vi "AddressGroup.vi"(11 "Addresses":i32[](array[numeric])=[0, 246, 248, 250]) -> (3 "Group":cluster{"Tag'sIndex":i32[]}[](array[cluster]))   [LabVIEW 2020, in "ModBusCommon.lvlib"]
uses:
  ModBusCommon.lvlib
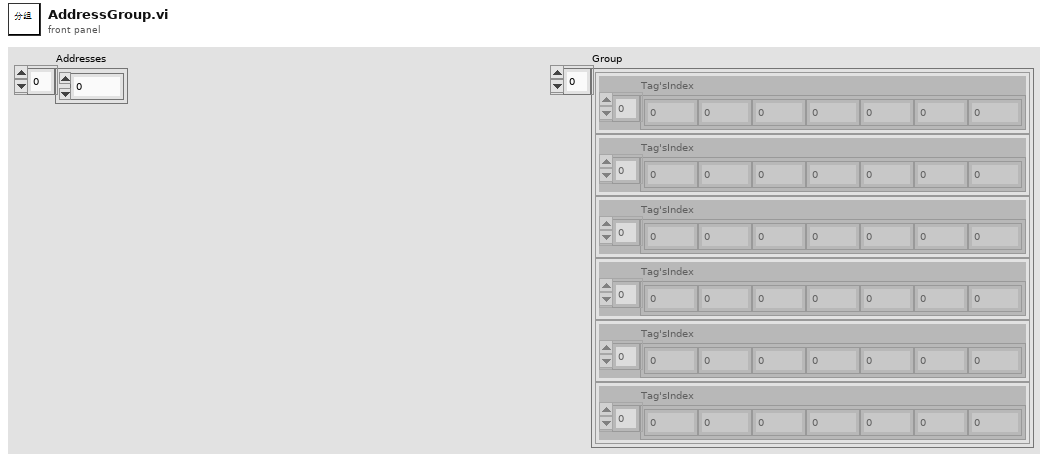
[diagram p1: front panel]
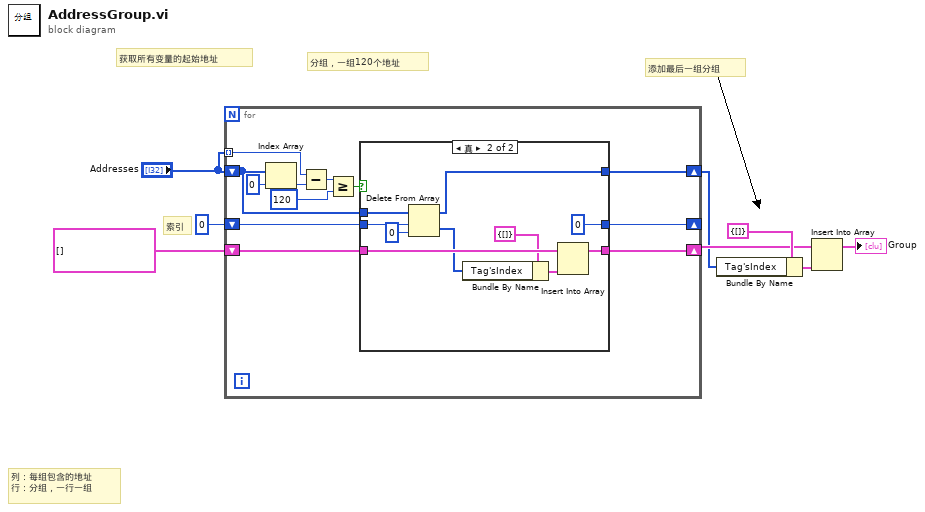
[diagram p0: block diagram]
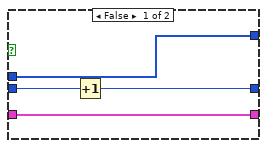
[diagram p2: hidden frame]
diagram:
  # "列：每组包含的地址\n行：分组，一行一组"
  # "添加最后一组分组"
  # "索引"
  # "分组，一组120个地址"
  # "获取所有变量的起始地址"
  n1 = for {
    tunnel: "Addresses" -> [w19] mode=indexing
    shift-right: [w11] -> w2
    shift-left: "Addresses" -> [w14]
    shift-right: [w12] -> _
    shift-left: 0 -> [w13]
    shift-right: [w9] -> w3
    shift-left: cluster{"Tag'sIndex":i32[]}[] [] -> [w10]
    n2 = Index Array(array=w14, index=0) -> (element=w18:i32)
    n3 = Subtract(x=w19, y=w18) -> (x-y=w17:i32)
    n4 = Greater Or Equal?(x=w17, y=120) -> (x >= y?=w15:bool)
    n5 = case shown="真" w15 {
      tunnel: w14 -> [w22 w34]
      tunnel: w13 -> [w24 w32]
      tunnel: [w23 0] -> w12
      tunnel: [w22 w30] -> w11
      tunnel: w10 -> [w21 w29]
      tunnel: [w21 w28] -> w9
      frame False {
        n6 = Increment(x=w24) -> (x+1=w23:i32)
      }
      frame True {
        n7 = Delete From Array(array=w34, length=w32, index=0) -> (deleted portion=w26:i32[], array with subset deleted=w30:i32[])
        n8 = Bundle By Name(cluster=cluster{"Tag'sIndex":i32[]} {"Tag'sIndex"=[]} ("Indexs"), "Tag'sIndex"=w26) -> (w25:cluster{"Tag'sIndex":i32[]})
        n9 = Insert Into Array(array=w29, new element=w25) -> (w28:cluster{"Tag'sIndex":i32[]}[])  [unwired: 1 in]
      }
    }
  }
  n10 = Bundle By Name(cluster=cluster{"Tag'sIndex":i32[]} {"Tag'sIndex"=[]} ("Indexs"), "Tag'sIndex"=w2) -> (w4:cluster{"Tag'sIndex":i32[]})
  n11 = Insert Into Array(array=w3, new element=w4) -> (→"Group":cluster{"Tag'sIndex":i32[]}[])  [unwired: 1 in]
